vi "Write Active Channel.vi"(8 "error in":errorcluster, 10 "Active Channel":u32, 11 "Electronic Load in":refnum<class "Electronic Load.lvclass">) -> (0 "error out":errorcluster, 3 "Electronic Load out":refnum<class "Electronic Load.lvclass">)   [LabVIEW 2019, in "Electronic Load.lvlib" / "Electronic Load.lvclass"]
uses:
  Library/Electronic Load.lvclass
  C:/Users/Public/Documents/Development/builds/Instruments/Instruments.lvlibp/Library/Instruments.lvclass
  Library/Electronic Load.lvclass/Electronic Load.ctl
  builds/Instruments/Instruments.lvlibp/Private/Polymorphic/Integers/Event from U32.vi
  builds/Instruments/Instruments.lvlibp/Accessors/Command with Logging.vi
  builds/Instruments/Instruments.lvlibp/Library/Instruments.lvclass
  builds/Instruments/Instruments.lvlibp
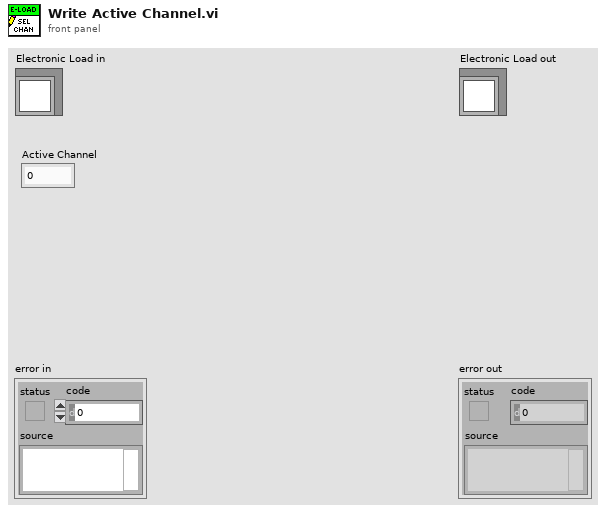
[diagram p1: front panel]
types:
  T1 = cluster{"Timestamp":timestamp, "Description":string, "Data":string}
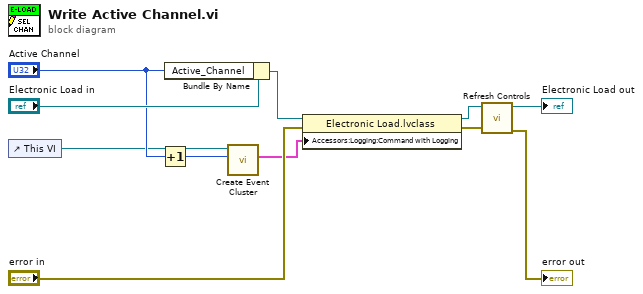
[diagram p0: block diagram]
diagram:
  n1 = control-ref of="This VI"() -> (w6:refnum<vi>)
  n2 = Increment(x="Active Channel") -> (x+1=w7:u32)
  n3 = Bundle By Name(cluster="Electronic Load in", "Active_Channel"="Active Channel") -> (w5:refnum<class "Electronic Load.lvclass">)
  n4 = call-poly "Create Event Cluster.vi"("Value"=w7, "VI Refnum"=w6) -> ("Event Data"=w1:T1)  [unwired: 9 in]
  n5 = property class="Electronic Load.lvclass"(reference=w5, error in="error in", "Accessors:Logging:Command with Logging"=w1) -> (reference out=w2:refnum<class "Electronic Load.lvclass">, error out=w4:errorcluster)
  n6 = call "Refresh Controls.vi"("error in"=w4, "Electronic Load in"=w2) -> ("error out"=→"error out":errorcluster, "Electronic Load out"=→"Electronic Load out":refnum<class "Electronic Load.lvclass">)  [unwired: 8 in]
